vi "OPC UA Secure Write Client2.vi"() -> ()   [LabVIEW 2017]
uses:
  <vilib>/OPCUA/controls/NodeId.ctl
  <vilib>/OPCUA/controls/Write Status.ctl
  <vilib>/OPCUA/client/Multiple Write Double.vi
  <vilib>/OPCUA/NI OPC UA Client.lvlib
panel:
  out "error out":errorcluster
  in  "requests":T3(array[cluster]) {"node status" items=["Good"=0, "Uncertain_InitialValue"=1083310080, "Uncertain_LastUsableValue"=1083179008, "Uncertain_SensorNotAccurate"=1083375616, "Uncertain_EngineeringUnitsExceeded"=1083441152, "Bad_NoCommunication"=2150694912, "Bad_NotReadable"=2151284736, "Bad_NotWritable"=2151350272, "Bad_OutOfRange"=2151415808, "Bad_WaitingForInitialData"=2150760448]}
  in  "stop":bool
  in  "trusted server certificates":path[](array[path])
  in  "client certificate file":path
  in  "server endpoint URL":string
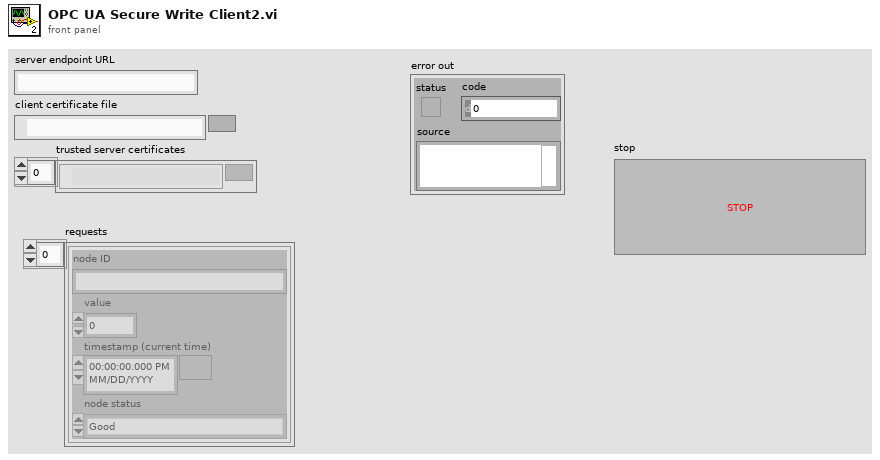
[diagram p1: front panel]
types:
  T1 = typedef "NodeId.ctl" = string
  T2 = typedef "Write Status.ctl" = u32
  T3 = cluster{"node ID":T1, "value":dbl, "timestamp (current time)":timestamp, "node status":T2}[]
  T4 = typedef "OPC UA Client Refnum.ctl" = refnum<k21>
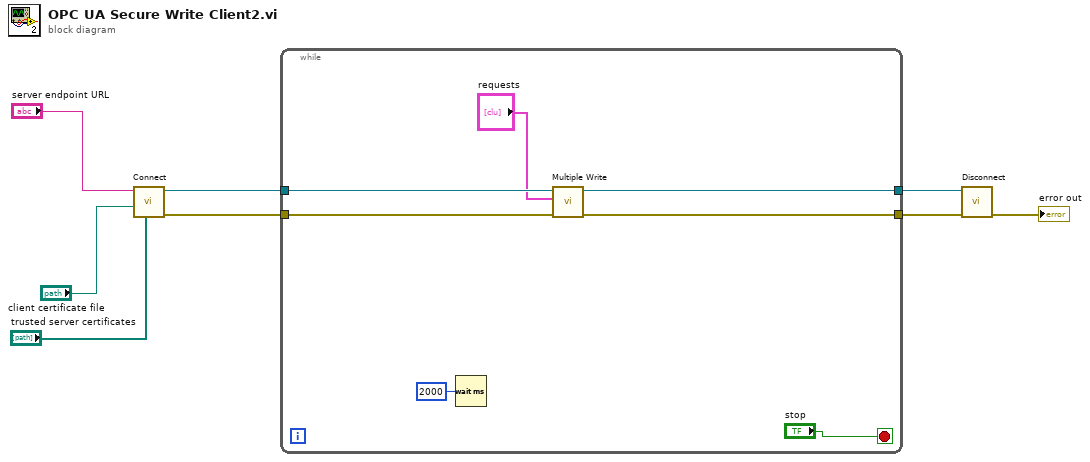
[diagram p0: block diagram]
diagram:
  n1 = call <vilib>:"Connect.vi"("trusted server certificates"="trusted server certificates", "client certificate file"="client certificate file", "server endpoint URL"="server endpoint URL") -> ("error out"=w3:errorcluster, "OPC UA client refnum out"=w5:T4)  [unwired: 6 in, 1 out]
  n2 = while {
    tunnel: w5 -> [w15]
    tunnel: [w14] -> w4
    tunnel: w3 -> [w13]
    tunnel: [w12] -> w2
    stop <- "stop" stop-if-true
    n3 = Wait (ms)(milliseconds to wait=u32 2000) -> ()  [unwired: 1 out]
    n4 = call-poly <vilib>:"Multiple Write.vi"("error in (no error)"=w13, "requests"="requests", "OPC UA client refnum in"=w15) -> ("error out"=w12:errorcluster, "OPC UA client refnum out"=w14:T4)  [unwired: 5 in, 2 out]
  }
  n5 = call <vilib>:"Disconnect.vi"("error in (no error)"=w2, "OPC UA client refnum in"=w4) -> ("error out"=→"error out":errorcluster)  [unwired: 9 in]
